vi "Insert_extra_rows_and_col.vi"(0 "Row Values In":dbl[](array[numeric]) format="%.2f", 1 "Additional Row Values":dbl[](array[numeric]) format="%.2f", 2 "Column Values In":dbl[](array[numeric]) format="%.2f", 3 "Data In":dbl[][](array[numeric]) format="%.2f", 4 "Additional Column Values":dbl[](array[numeric]) format="%.2f") -> (6 "Row Values Out":dbl[](array[numeric]) format="%.2f", 7 "Column Values Out":dbl[](array[numeric]) format="%.2f", 9 "Data Out":dbl[][](array[numeric]) format="%.2f")   [LabVIEW 2020]
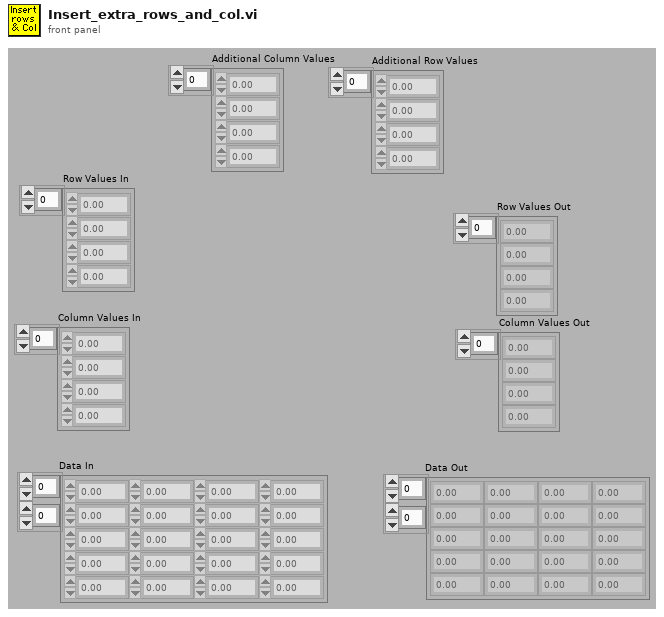
[diagram p1: front panel]
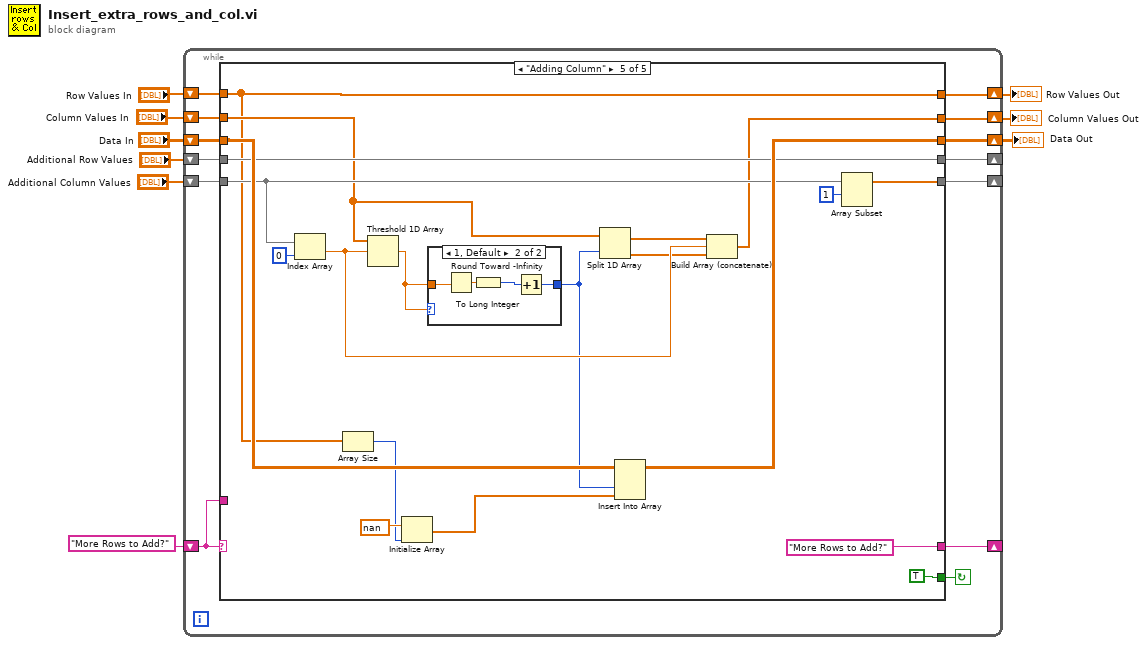
[diagram p0: block diagram]
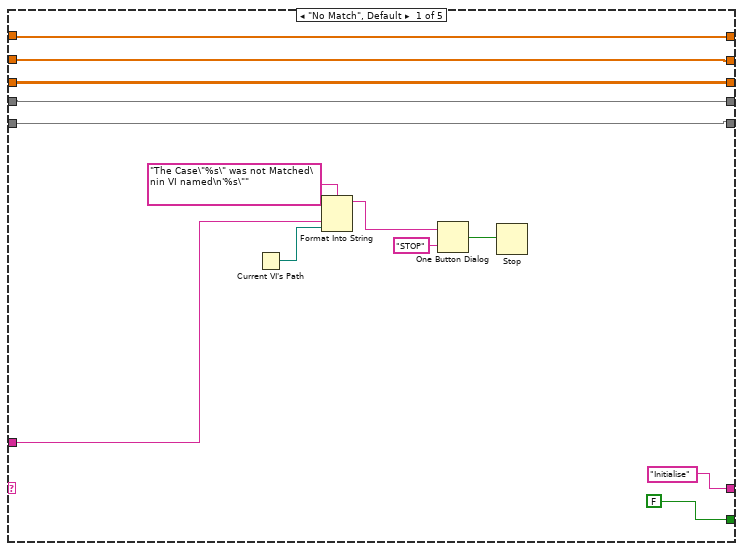
[diagram p2: hidden frame]
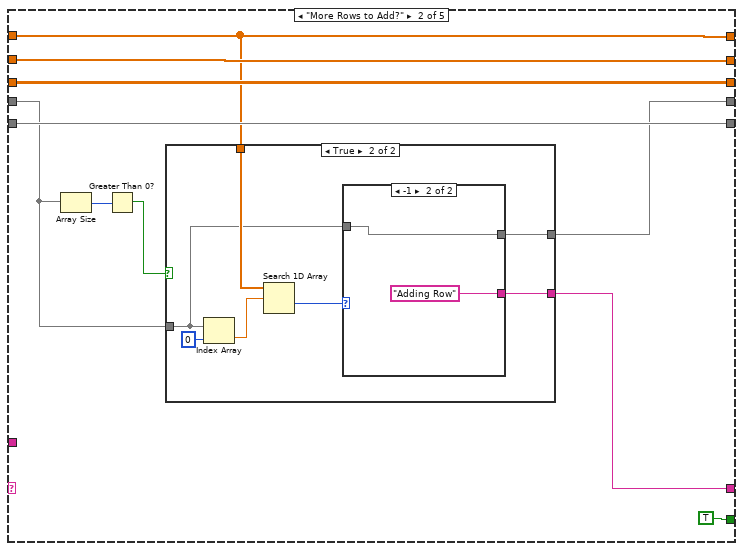
[diagram p3: hidden frame]
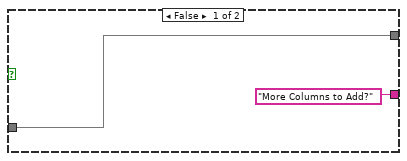
[diagram p4: hidden frame]
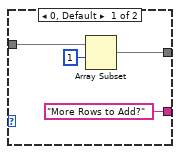
[diagram p5: hidden frame]
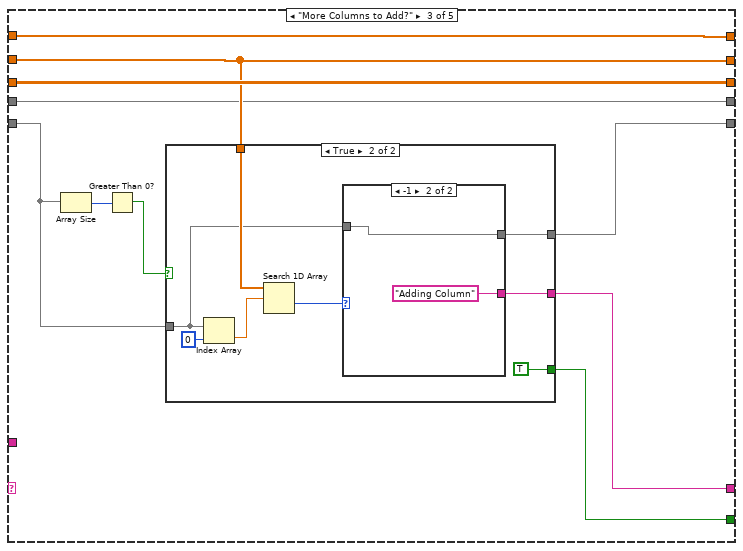
[diagram p6: hidden frame]
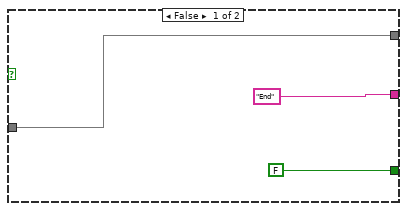
[diagram p7: hidden frame]
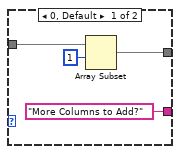
[diagram p8: hidden frame]
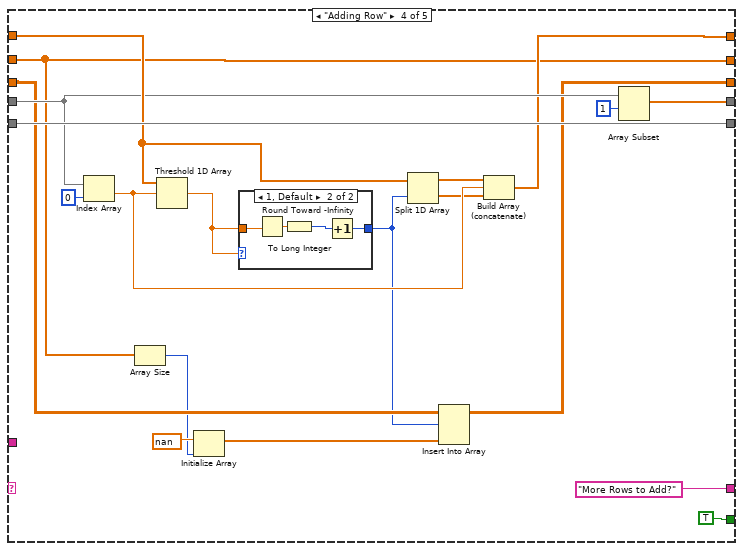
[diagram p9: hidden frame]
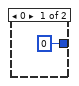
[diagram p10: hidden frame]
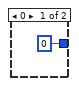
[diagram p11: hidden frame]
diagram:
  n1 = while {
    shift-left: "More Rows to Add?" -> [w20]
    shift-right: [w21] -> _
    shift-right: [w19] -> w3
    shift-left: "Row Values In" -> [w18]
    shift-right: [w17] -> w4
    shift-left: "Column Values In" -> [w16]
    shift-right: [w15] -> w5
    shift-left: "Data In" -> [w14]
    shift-right: [w12] -> _
    shift-left: "Additional Row Values" -> [w13]
    shift-right: [w11] -> _
    shift-left: "Additional Column Values" -> [w10]
    stop <- w22 continue-if-true
    n2 = case shown="\"Adding Column\"" w20 {
      tunnel: [FALSE TRUE w66 TRUE TRUE] -> w22
      tunnel: ["Initialise" w38 w67 "More Rows to Add?" "More Rows to Add?"] -> w21
      tunnel: w20 -> [w30 _ _ _ _]
      tunnel: [w27 w39 w65 w97 w116] -> w19
      tunnel: w18 -> [w27 w39 w65 w101 w116]
      tunnel: [w26 w44 w64 w91 w120] -> w17
      tunnel: w16 -> [w26 w44 w64 w91 w121]
      tunnel: [w25 w43 w70 w94 w125] -> w15
      tunnel: w14 -> [w25 w43 w70 w95 w126]
      tunnel: w13 -> [w24 w37 w63 w100 w123]
      tunnel: [w24 w36 w63 w98 w123] -> w12
      tunnel: [w23 w42 w62 w106 w124] -> w11
      tunnel: w10 -> [w23 w42 w61 w106 w122]
      frame "No Match", Default {
        n3 = Current VI's Path() -> (path=w29:path)
        n4 = Format Into String(format string="The Case\"%s\" was not Matched\nin VI named\n'%s\"" ("Format String"), w30, w29) -> (resulting string=w33:string)  [unwired: 2 in, 1 out]
        n5 = One Button Dialog(message=w33, button name ("OK")="STOP") -> (true=w31:bool)
        n6 = Stop(stop? (T)=w31) -> ()
      }
      frame "More Rows to Add?" {
        n7 = Array Size(array=w37) -> (size(s)=w41:i32)
        n8 = Greater Than 0?(x=w41) -> (x > 0?=w40:bool)
        n9 = case shown="True" w40 {
          tunnel: w37 -> [w46 w49]
          tunnel: w39 -> [_ w53]
          tunnel: ["More Columns to Add?" w50] -> w38
          tunnel: [w46 w48] -> w36
          frame False {
          }
          frame True {
            n10 = Index Array(array=w49, index=0) -> (element=w52:dbl)
            n11 = Search 1D Array(1D array=w53, element=w52) -> (index of element=w51:i32)  [unwired: 1 out]
            n12 = case shown="-1" w51 {
              tunnel: ["More Rows to Add?" "Adding Row"] -> w50
              tunnel: w49 -> [w56 w59]
              tunnel: [w55 w59] -> w48
              frame 0, Default {
                n13 = Array Subset(array=w56, index=1) -> (w55:dbl[])  [unwired: 1 in]
              }
              frame -1 {
              }
            }
          }
        }
      }
      frame "More Columns to Add?" {
        n14 = Array Size(array=w61) -> (size(s)=w69:i32)
        n15 = Greater Than 0?(x=w69) -> (x > 0?=w68:bool)
        n16 = case shown="True" w68 {
          tunnel: w61 -> [w72 w76]
          tunnel: w64 -> [_ w80]
          tunnel: ["End" w77] -> w67
          tunnel: [w72 w75] -> w62
          tunnel: [FALSE TRUE] -> w66
          frame False {
          }
          frame True {
            n17 = Index Array(array=w76, index=0) -> (element=w79:dbl)
            n18 = Search 1D Array(1D array=w80, element=w79) -> (index of element=w78:i32)  [unwired: 1 out]
            n19 = case shown="-1" w78 {
              tunnel: ["More Columns to Add?" "Adding Column"] -> w77
              tunnel: w76 -> [w83 w86]
              tunnel: [w82 w86] -> w75
              frame 0, Default {
                n20 = Array Subset(array=w83, index=1) -> (w82:dbl[])  [unwired: 1 in]
              }
              frame -1 {
              }
            }
          }
        }
      }
      frame "Adding Row" {
        n21 = Index Array(array=w100, index=0) -> (element=w103:dbl)
        n22 = Array Size(array=w91) -> (size(s)=w90:i32)
        n23 = Threshold 1D Array(2:w103, 3:w101) -> (0:w88:dbl)  [unwired: 1 out]
        n24 = Initialize Array(nan, w90) -> (w92:dbl[])
        n25 = case shown="1, Default" w88 {
          tunnel: w88 -> [_ w112]
          tunnel: [0 w109] -> w89
          frame 0 {
          }
          frame 1, Default {
            n26 = Round Toward -Infinity(1:w112) -> (0:w111:dbl)
            n27 = To Long Integer(number=w111) -> (32bit integer=w110:i32)
            n28 = Increment(x=w110) -> (x+1=w109:i32)
          }
        }
        n29 = Split 1D Array(array=w101, index=w89) -> (first subarray=w104:dbl[], second subarray=w102:dbl[])
        n30 = Insert Into Array(array=w95, index (row)=w89, new element=w92) -> (w94:dbl[][])  [unwired: 1 in]
        n31 = Build Array (concatenate)(w104, w103, w102) -> (w97:dbl[])
        n32 = Array Subset(array=w100, index=1) -> (w98:dbl[])  [unwired: 1 in]
      }
      frame "Adding Column" {
        n33 = Index Array(array=w122, index=0) -> (element=w130:dbl)
        n34 = Array Size(array=w116) -> (size(s)=w118:i32)
        n35 = Threshold 1D Array(2:w130, 3:w121) -> (0:w113:dbl)  [unwired: 1 out]
        n36 = Initialize Array(nan, w118) -> (w117:dbl[])
        n37 = case shown="1, Default" w113 {
          tunnel: w113 -> [_ w137]
          tunnel: [0 w134] -> w115
          frame 0 {
          }
          frame 1, Default {
            n38 = Round Toward -Infinity(1:w137) -> (0:w136:dbl)
            n39 = To Long Integer(number=w136) -> (32bit integer=w135:i32)
            n40 = Increment(x=w135) -> (x+1=w134:i32)
          }
        }
        n41 = Split 1D Array(array=w121, index=w115) -> (first subarray=w114:dbl[], second subarray=w129:dbl[])
        n42 = Insert Into Array(array=w126, index (col)=w115, new element=w117) -> (w125:dbl[][])  [unwired: 1 in]
        n43 = Build Array (concatenate)(w114, w130, w129) -> (w120:dbl[])
        n44 = Array Subset(array=w122, index=1) -> (w124:dbl[])  [unwired: 1 in]
      }
    }
  }
  "Row Values Out" <- w3
  "Column Values Out" <- w4
  "Data Out" <- w5
